vi "RT_Loop_junk.vi"(0 "PXI card names":string[](array[string])=["DIO:", "6509", "Counter:", "6733_1", "Slow AO:", "6723", "Fast AO:", "6733_1", "6733_2"], 1 "Param Qname":T1, 2 "RT Loop Qname":T1, 3 "Handler Qname":T1) -> ()   [LabVIEW 2018]
uses:
  <vilib>/NI/AMC/Message Queue.ctl
  <vilib>/NI/AMC/Message.ctl
  <vilib>/NI/Tools/Keyed Array/KeyedArray.ctl
  RT_State.ctl
  <vilib>/Utility/error.llb/DialogType.ctl
  ActionCluster.ctl
  Instructions_RT.ctl
  ParameterSubCluster.ctl
  Request.ctl
  <vilib>/DAQmx/read.llb/DAQmx Read (Digital 1D Bool NChan 1Samp 1Line).vi
  <vilib>/NI/AMC/Read Termination Message.vi
  <vilib>/NI/AMC/Create Single Message.vi
  <vilib>/NI/AMC/Update Message Routing Info.vi
  <vilib>/NI/AMC/Globals.vi
  <vilib>/NI/AMC/Send Message.vi
  <vilib>/DAQmx/miscellaneous.llb/DAQmx Fill In Error Info.vi
  <vilib>/NI/AMC/AMC.lvlib
  <vilib>/NI/Tools/Keyed Array/Tools_KeyedArray.lvlib
panel:
  in  "min Action time (s)":dbl=0.01 format="%#_13g"
  in  "max Action time (s)":dbl=1000.0 format="%#_13g"
  out "error out":errorcluster
  in  "stop RT loop":bool
  out "Action #":i32=14
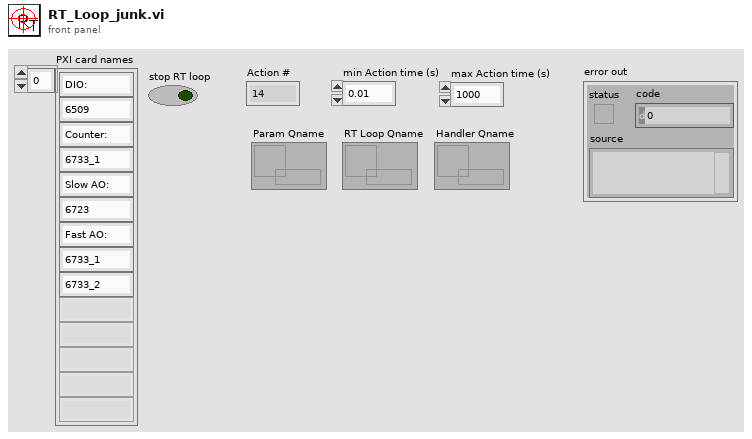
[diagram p1: front panel]
types:
  T1 = typedef "AMC.lvlib/Message Queue.ctl" = refnum<queue>
  T2 = typedef "ActionCluster.ctl" = cluster{"Macro Instructions":T3, "Slow AO Array":T4, "Duration (s)":dbl, "Toggle":bool}
  T3 = typedef "Instructions_RT.ctl" = cluster{"Duration (s)":dbl, "Steps":i32, "Changes":bool[], "Triggers":bool[], "RAW cmds 2D":i16[][]}[]
  T4 = typedef "ParameterSubCluster.ctl" = cluster{"ao line":string, "Duration, Gain, NewVal":dbl[]}[]
  T5 = typedef "DialogType.ctl" = u16
  T6 = typedef "RT_State.ctl" = enum16{"Idle", "Run", "Macro", "Param", "Inbit"}
  T7 = typedef "Tasks_RT.ctl" = cluster{"inbits":i32, "outbits":i32, "Counter":refnum<k21>, "Inbits":refnum<k21>, "Outbits":refnum<k21>, "Fast AO":refnum<k21>[], "Errors":errorcluster}
  T8 = typedef "Request.ctl" = enum16{"New Cue", "Run", "Skip Wait", "Pause", "Unpause", "Abort", "Shutdown"}
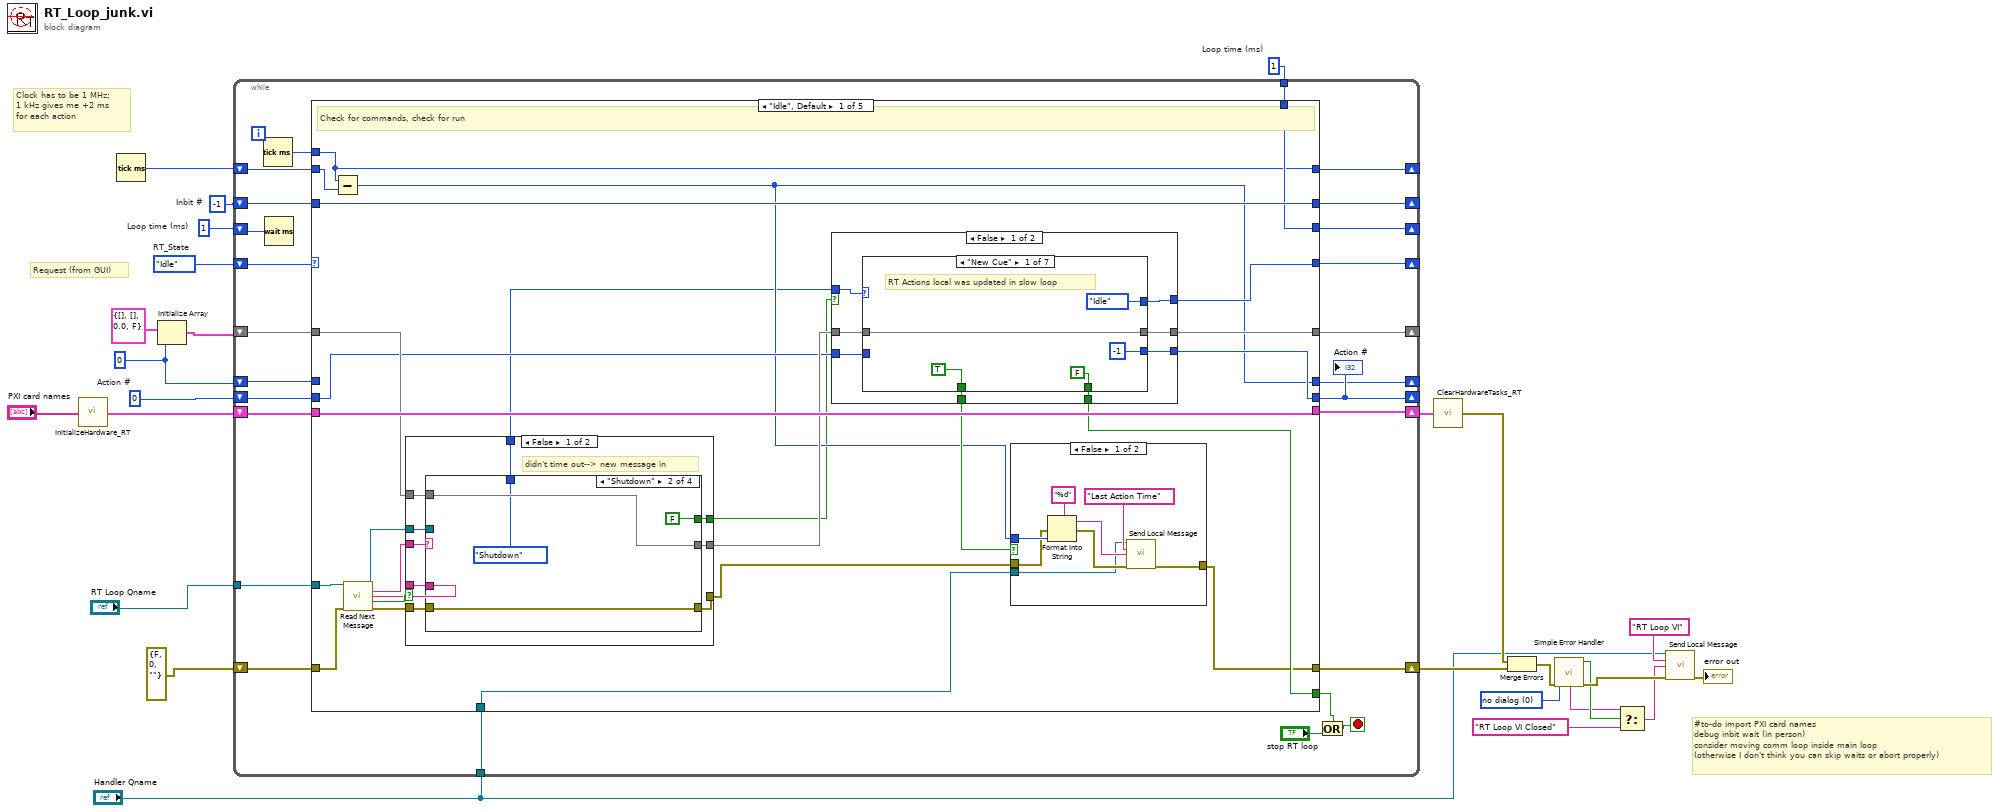
[diagram p0: block diagram]
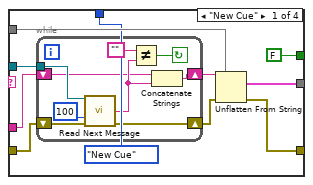
[diagram p3: hidden frame]
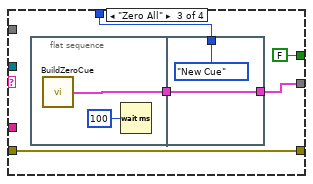
[diagram p4: hidden frame]
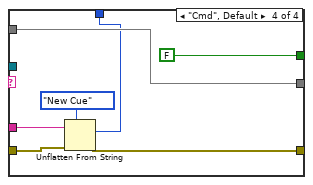
[diagram p5: hidden frame]
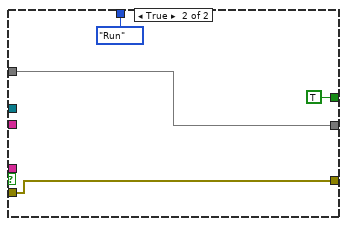
[diagram p6: hidden frame]
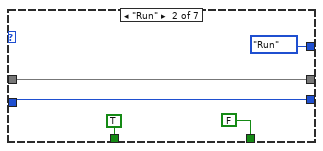
[diagram p7: hidden frame]
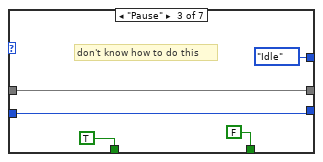
[diagram p8: hidden frame]
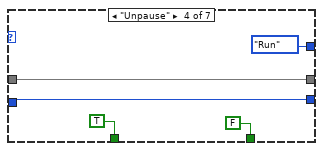
[diagram p9: hidden frame]
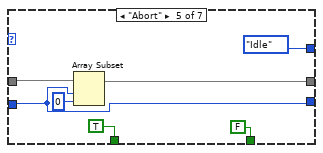
[diagram p10: hidden frame]
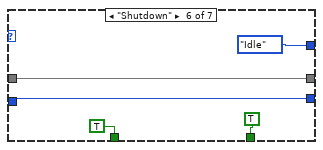
[diagram p11: hidden frame]
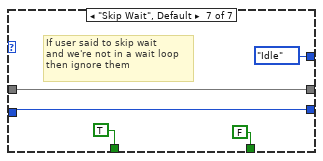
[diagram p12: hidden frame]
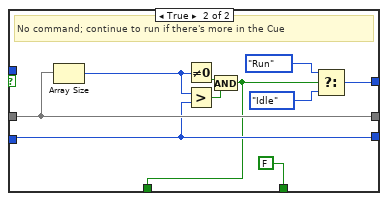
[diagram p13: hidden frame]
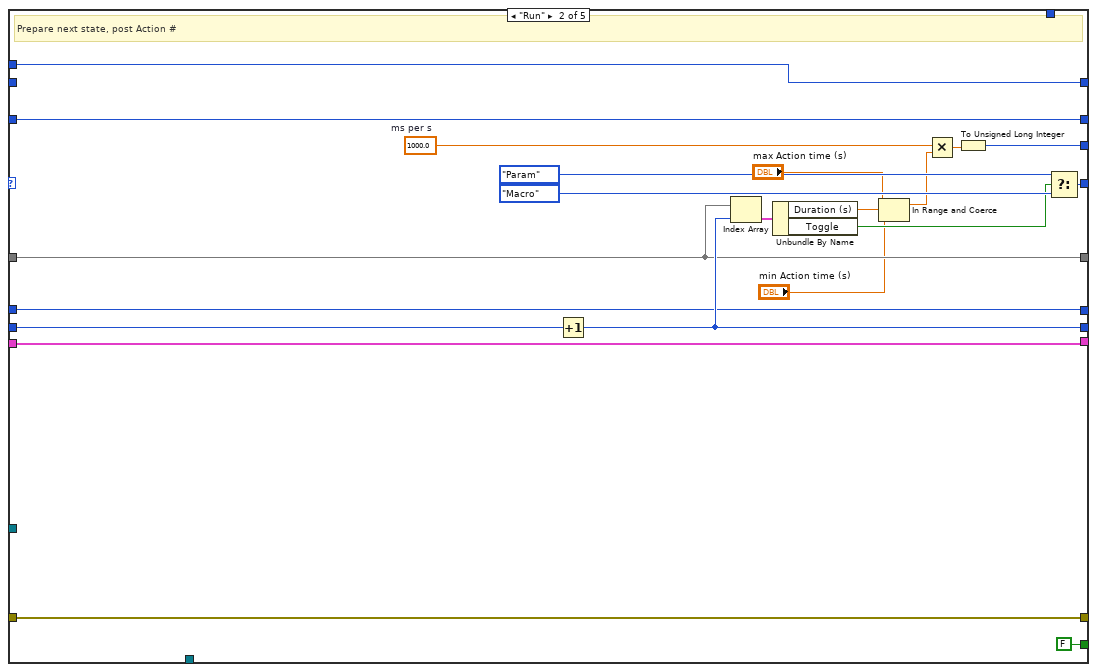
[diagram p14: hidden frame]
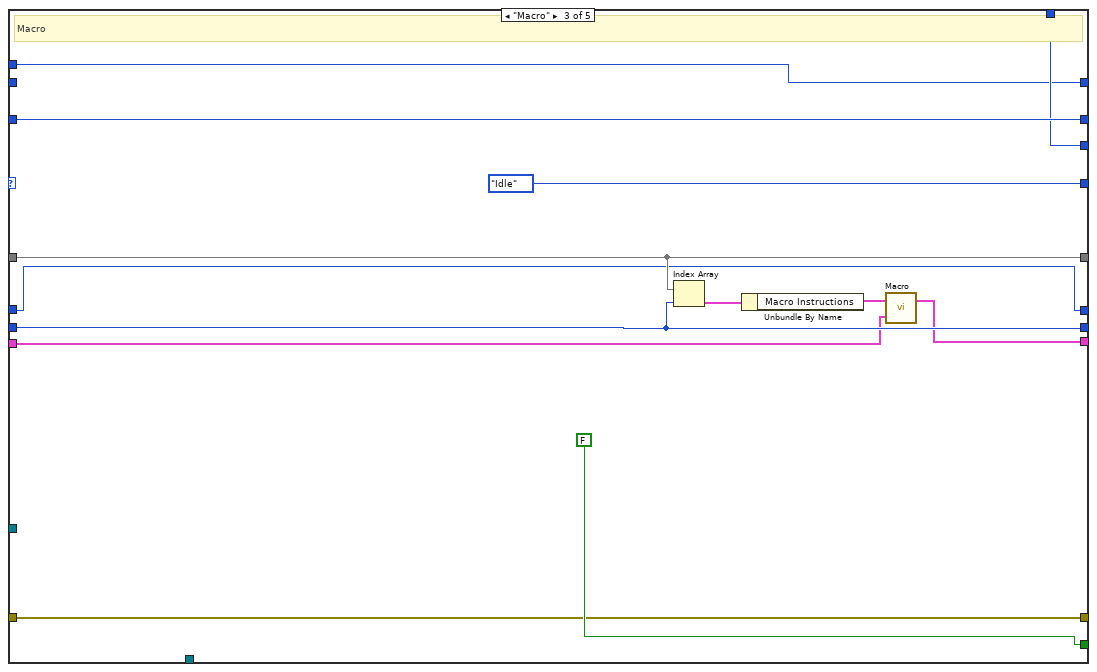
[diagram p15: hidden frame]
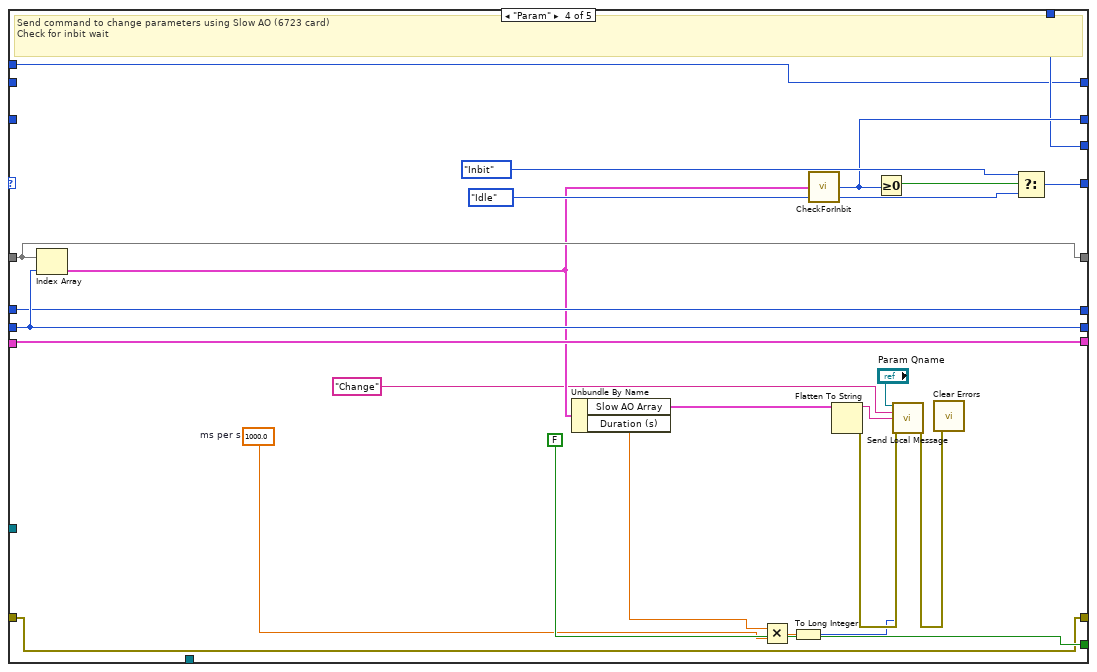
[diagram p16: hidden frame]
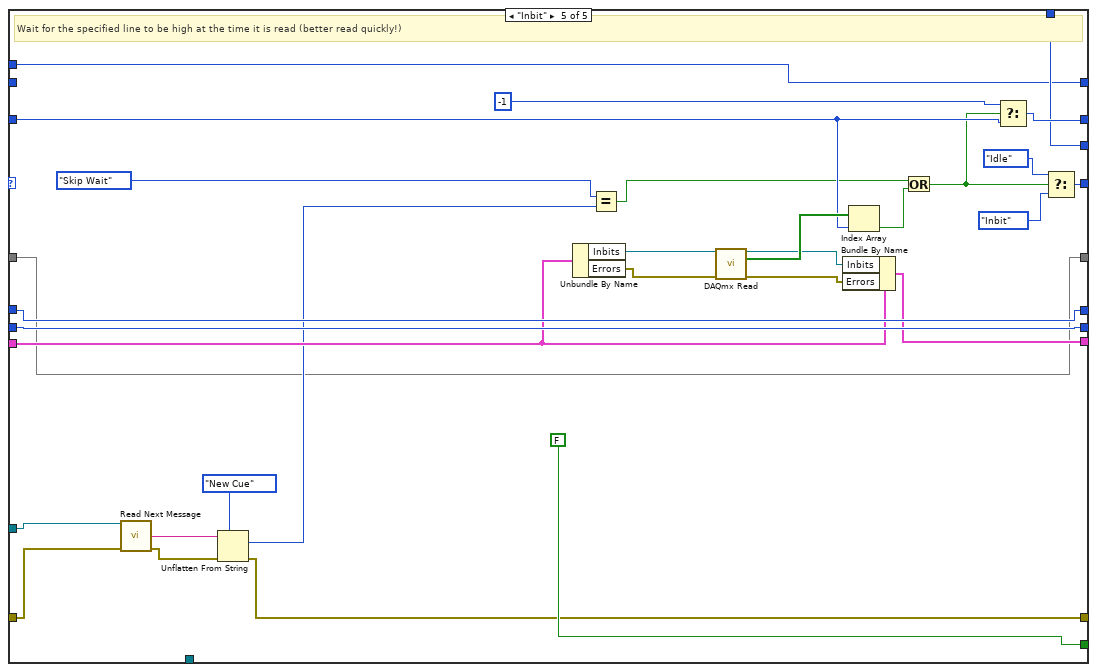
[diagram p17: hidden frame]
diagram:
  w7 = u32 1  # Loop time (ms)
  w9 = u32 1  # Loop time (ms)
  w6 = u32 0 ("dimension size")
  w18 = T5 0 items=["no dialog", "OK message", "continue or stop message", "OK message + warnings", "continue/stop + warnings"] ("type of dialog (OK msg:1)")
  w20 = -1  # Inbit #
  w22 = RT_State."Idle"  # RT_State
  w23 = 0  # Action #
  # "#to-do import PXI card names\ndebug inbit wait (in person)\nconsider moving comm loop inside main loop\n(otherwise I don't think you can skip waits or abort properly)"
  # "Clock has to be 1 MHz;\n1 kHz gives me +2 ms\nfor each action"
  # "Request (from GUI)"
  n1 = call "InitializeHardware_RT.vi"("PXI card names"="PXI card names") -> ("Task cluster"=w24:T7)
  n2 = Tick Count (ms)() -> (millisecond timer value=w8:u32)
  n3 = Initialize Array(T2 {"Macro Instructions"=[], "Slow AO Array"=[], "Duration (s)"=0.0, "Toggle"=FALSE} ("element"), w6) -> (w10:T2[])
  n4 = while {
    shift-right: [w50] -> _
    shift-left: w22 -> [w51]
    shift-right: [w47] -> _
    shift-left: w23 -> [w48]
    shift-right: [w46] -> _
    shift-left: w20 -> [w45]
    shift-right: [w44] -> _
    shift-left: w10 -> [w49]
    shift-right: [w42] -> w26
    shift-left: w24 -> [w43]
    shift-right: [w38] -> _
    shift-left: w6 -> [w37]
    shift-right: [w36] -> _
    shift-left: w9 -> [w35]
    shift-right: [w31] -> _
    shift-left: w8 -> [w32]
    tunnel: w7 -> [w34]
    shift-right: [w29] -> w3
    shift-left: errorcluster {"status"=FALSE, "code"=0, "source"=""} ("error out") -> [w30]
    tunnel: "Handler Qname" -> [w28]
    tunnel: "RT Loop Qname" -> [w27]
    stop <- w41 stop-if-true
    n5 = Tick Count (ms)() -> (millisecond timer value=w33:u32)
    n6 = Wait (ms)(milliseconds to wait=w35) -> ()  [unwired: 1 out]
    n7 = case shown="\"Idle\", Default" w51 {
      tunnel: [w76 w214 RT_State."Idle" ("RT_State") w248 w275] -> w50
      tunnel: [w71 w213 w217 w230 w266] -> w36
      tunnel: [w73 FALSE FALSE FALSE FALSE] -> w40
      tunnel: w49 -> [w63 w205 w223 w241 w252]
      tunnel: w48 -> [w59 w198 w225 w250 w280]
      tunnel: [w72 w211 w225 w250 w280] -> w47
      tunnel: [w77 w212 w224 w245 w271] -> w46
      tunnel: w45 -> [w77 w212 w224 _ w273]
      tunnel: [w75 w205 w223 w241 w252] -> w44
      tunnel: w43 -> [w74 w204 w222 w244 w263]
      tunnel: [w74 w204 w221 w244 w261] -> w42
      tunnel: [w54 w196 w218 w243 w267] -> w38
      tunnel: w37 -> [_ w196 w218 w243 w267]
      tunnel: w34 -> [w71 _ w217 w230 w266]
      tunnel: w33 -> [w69 w197 w216 w229 w265]
      tunnel: w32 -> [w70 _ _ _ _]
      tunnel: [w69 w197 w216 w229 w265] -> w31
      tunnel: w30 -> [w62 w194 w215 w228 w259]
      tunnel: [w56 w194 w215 w228 w255] -> w29
      tunnel: w28 -> [w55 _ _ _ _]
      tunnel: w27 -> [w61 _ _ _ w253]
      frame "Idle", Default {
        # "Check for commands, check for run"
        n8 = Subtract(x=w69, y=w70) -> (x-y=w54:u32)
        n9 = call <vilib>:"Read Next Message.vi"("message queue in"=w61, "error in"=w62) -> ("message queue out"=w68:T1, "message name"=w67:string, "message value"=w64:string, "timed out?"=w65:bool, "error out"=w66:errorcluster)  [unwired: 6 in, 3 out]
        n10 = case shown="False" w65 {
          tunnel: w64 -> [w95 _]
          tunnel: [w94 w136] -> w58
          tunnel: w66 -> [w93 w136]
          tunnel: w67 -> [w92 _]
          tunnel: [w91 TRUE] -> w53
          tunnel: w68 -> [w90 _]
          tunnel: [w89 w137] -> w60
          tunnel: w63 -> [w88 w137]
          tunnel: [w87 Request."Run" ("RT_State")] -> w52
          frame False {
            # "didn't time out--> new message in"
            n11 = case shown="\"Shutdown\"" w92 {
              tunnel: w95 -> [w97 _ _ w134]
              tunnel: [w100 w117 w122 w128] -> w94
              tunnel: w93 -> [w103 w117 w122 w133]
              tunnel: [FALSE FALSE FALSE FALSE] -> w91
              tunnel: w90 -> [w104 _ _ _]
              tunnel: [w99 w116 w121 w130] -> w89
              tunnel: w88 -> [w98 w116 _ w130]
              tunnel: [Request."New Cue" ("RT_State") Request."Shutdown" ("RT_State") w119 w129] -> w87
              frame "New Cue" {
                n12 = while {
                  tunnel: w104 -> [w114]
                  shift-right: [w111] -> w101
                  shift-left: w103 -> [w112]
                  shift-right: [w109] -> w102
                  shift-left: w97 -> [w108]
                  stop <- w106 continue-if-true
                  n13 = call <vilib>:"Read Next Message.vi"("message queue in"=w114, "timeout (1 ms)"=100, "error in"=w112) -> ("message value"=w110:string, "error out"=w111:errorcluster)  [unwired: 5 in, 6 out]
                  n14 = Not Equal?(x="", y=w110) -> (x != y?=w106:bool)
                  n15 = Concatenate Strings(w108, w110) -> (w109:string)
                }
                n16 = Unflatten From String(type=w98, binary string=w102, error in (no error)=w101) -> (value=w99:T2[], error out=w100:errorcluster)  [unwired: 2 in, 1 out]
              }
              frame "Shutdown" {
              }
              frame "Zero All" {
                n17 = flat-sequence {
                  tunnel: [w125] -> w120
                  tunnel: [w127] -> w121
                  tunnel: w120 -> [w127]
                  tunnel: [Request."New Cue" ("RT_State")] -> w119
                  frame #0 {
                    n18 = call "BuildZeroCue.vi"() -> ("Zero Cue"=w125:T2[])  [unwired: 3 in]
                    n19 = Wait (ms)(milliseconds to wait=u32 100) -> ()  [unwired: 1 out]
                  }
                  frame #1 {
                  }
                }
              }
              frame "Cmd", Default {
                n20 = Unflatten From String(type=Request."New Cue" ("RT_State"), binary string=w134, error in (no error)=w133) -> (value=w129:T8, error out=w128:errorcluster)  [unwired: 2 in, 1 out]
              }
            }
          }
          frame True {
          }
        }
        n21 = case shown="False" w53 {
          tunnel: w60 -> [w144 w187]
          tunnel: w59 -> [w143 w185]
          tunnel: [w146 w188] -> w76
          tunnel: [w145 w187] -> w75
          tunnel: [w142 FALSE] -> w73
          tunnel: [w141 w185] -> w72
          tunnel: [w140 w184] -> w57
          tunnel: w52 -> [w139 _]
          frame False {
            n22 = case shown="\"New Cue\"" w139 {
              tunnel: [RT_State."Idle" ("RT_State") RT_State."Run" ("RT_State") RT_State."Idle" ("RT_State") RT_State."Run" ("RT_State") RT_State."Idle" ("RT_State") RT_State."Idle" ("RT_State") RT_State."Idle" ("RT_State")] -> w146
              tunnel: [w147 w155 w161 w166 w171 w176 w183] -> w145
              tunnel: w144 -> [w147 w155 w161 w166 w172 w176 w183]
              tunnel: w143 -> [_ w153 w158 w163 w168 w175 w180]
              tunnel: [FALSE FALSE FALSE FALSE FALSE TRUE FALSE] -> w142
              tunnel: [-1 w153 w158 w163 w168 w175 w180] -> w141
              tunnel: [TRUE TRUE TRUE TRUE TRUE TRUE TRUE] -> w140
              frame "New Cue" {
                # "RT Actions local was updated in slow loop"
              }
              frame "Run" {
              }
              frame "Pause" {
                # "don't know how to do this"
              }
              frame "Unpause" {
              }
              frame "Abort" {
                n23 = Array Subset(array=w172, index=w168, length=0) -> (w171:T2[])
              }
              frame "Shutdown" {
              }
              frame "Skip Wait", Default {
                # "If user said to skip wait\nand we're not in a wait loop\nthen ignore them"
              }
            }
          }
          frame True {
            # "No command; continue to run if there's more in the Cue"
            n24 = Array Size(array=w187) -> (size(s)=w193:i32)
            n25 = Not Equal To 0?(x=w193) -> (x != 0?=w192:bool)
            n26 = Greater?(x=w193, y=w185) -> (0:w191:bool)
            n27 = And(x=w192, y=w191) -> (x .and. y?=w184:bool)
            n28 = Select(t=RT_State."Run" ("RT_State"), s=w184, f=RT_State."Idle" ("RT_State")) -> (s? t:f=w188:T6)
          }
        }
        n29 = case shown="False" w57 {
          tunnel: w55 -> [w78 _]
          tunnel: w54 -> [w81 _]
          tunnel: [w84 w86] -> w56
          tunnel: w58 -> [w79 w86]
          frame False {
            n30 = Format Into String(format string="%d", error in=w79, w81) -> (resulting string=w82:string, error out=w83:errorcluster)  [unwired: 1 in]
            n31 = call <vilib>:"Send Local Message.vi"("message queue in"=w78, "message name"="Last Action Time", "message value"=w82, "error in"=w83) -> ("error out"=w84:errorcluster)  [unwired: 9 in, 2 out]
          }
          frame True {
            # "no new Action"
          }
        }
      }
      frame "Run" {
        w208 = 1000.0  # ms per s
        # "Prepare next state, post Action #"
        n32 = Increment(x=w198) -> (x+1=w211:i32)
        n33 = Index Array(array=w205, index=w211) -> (element=w207:T2)
        n34 = Unbundle By Name(w207) -> ("Duration (s)"=w203:dbl, "Toggle"=w206:bool)
        n35 = In Range and Coerce(upper limit="max Action time (s)", x=w203, lower limit="min Action time (s)") -> (coerced(x)=w199:dbl)  [unwired: 1 out]
        n36 = Multiply(x=w208, y=w199) -> (x*y=w200:dbl)
        n37 = To Unsigned Long Integer(number=w200) -> (unsigned 32bit integer=w213:u32)
        n38 = Select(t=RT_State."Param" ("RT_State"), s=w206, f=RT_State."Macro" ("RT_State")) -> (s? t:f=w214:T6)
      }
      frame "Macro" {
        # "Macro"
        n39 = Index Array(array=w223, index=w225) -> (element=w219:T2)
        n40 = Unbundle By Name(w219) -> ("Macro Instructions"=w220:T3)
        n41 = call "Macro.vi"("Tasks in"=w222, "Macro Instructions"=w220) -> ("Tasks out"=w221:T7)  [unwired: 1 in]
      }
      frame "Param" {
        w233 = 1000.0  # ms per s
        # "Send command to change parameters using Slow AO (6723 card)\nCheck for inbit wait"
        n42 = Index Array(array=w241, index=w250) -> (element=w240:T2)
        n43 = Unbundle By Name(w240) -> ("Slow AO Array"=w242:T4, "Duration (s)"=w234:dbl)
        n44 = Multiply(x=w234, y=w233) -> (x*y=w232:dbl)
        n45 = To Long Integer(number=w232) -> (32bit integer=w231:i32)
        n46 = call "CheckForInbit.vi"("Action"=w240) -> ("Inbit #"=w245:i32)
        n47 = Flatten To String(anything=w242) -> (data string=w239:string, error out=w238:errorcluster)  [unwired: 3 in, 1 out]
        n48 = Greater Or Equal To 0?(x=w245) -> (x >= 0?=w246:bool)
        n49 = call <vilib>:"Send Local Message.vi"("message queue in"="Param Qname", "message name"="Change", "message value"=w239, "timeout (-1 ms)"=w231, "error in"=w238) -> ("error out"=w236:errorcluster)  [unwired: 8 in, 2 out]
        n50 = call <vilib>:"Clear Errors.vi"("error in (no error)"=w236) -> ()  [unwired: 5 in, 2 out]
        n51 = Select(t=RT_State."Inbit" ("RT_State"), s=w246, f=RT_State."Idle" ("RT_State")) -> (s? t:f=w248:T6)
      }
      frame "Inbit" {
        # "Wait for the specified line to be high at the time it is read (better read quickly!)"
        n52 = call <vilib>:"Read Next Message.vi"("message queue in"=w253, "error in"=w259) -> ("message value"=w258:string, "error out"=w256:errorcluster)  [unwired: 6 in, 6 out]
        n53 = Unflatten From String(type=Request."New Cue" ("RT_State"), binary string=w258, error in (no error)=w256) -> (value=w254:T8, error out=w255:errorcluster)  [unwired: 2 in, 1 out]
        n54 = Unbundle By Name(w263) -> ("Inbits"=w279:refnum<k21>, "Errors"=w264:errorcluster)
        n55 = Equal?(x=Request."Skip Wait" ("RT_State"), y=w254) -> (x = y?=w268:bool)
        n56 = call-poly <vilib>:"DAQmx Read.vi"("task/channels in"=w279, "error in"=w264) -> ("task out"=w260:refnum<k21>, "data"=w278:bool[], "error out"=w262:errorcluster)  [unwired: 11 in]
        n57 = Bundle By Name(cluster=w263, "Inbits"=w260, "Errors"=w262) -> (w261:T7)
        n58 = Index Array(array=w278, index=w273) -> (element=w269:bool)
        n59 = Or(x=w268, y=w269) -> (x .or. y?=w270:bool)
        n60 = Select(t=-1, s=w270, f=w273) -> (s? t:f=w271:i32)
        n61 = Select(t=RT_State."Idle" ("RT_State"), s=w270, f=RT_State."Inbit" ("RT_State")) -> (s? t:f=w275:T6)
      }
    }
    "Action #" <- w47
    n62 = Or(x=w40, y="stop RT loop") -> (x .or. y?=w41:bool)
  }
  n63 = call "ClearHardwareTasks_RT.vi"("Task cluster"=w26) -> ("Errors"=w5:errorcluster)
  n64 = Merge Errors(w5, w3) -> (w19:errorcluster)
  n65 = call <vilib>:"Simple Error Handler.vi"("type of dialog (OK msg:1)"=w18, "error in (no error)"=w19) -> ("error?"=w15:bool, "error out"=w17:errorcluster, "message"=w14:string)  [unwired: 3 in, 2 out]
  n66 = Select(t=w14, s=w15, f="RT Loop VI Closed" ("message name")) -> (s? t:f=w13:string)
  n67 = call <vilib>:"Send Local Message.vi"("message queue in"="Handler Qname", "message name"="RT Loop VI", "message value"=w13, "error in"=w17) -> ("error out"=→"error out":errorcluster)  [unwired: 9 in, 2 out]
